vi "ISEG_HVBoardGUI.getStatus.vi"(2 "Numeric":dbl) -> (16 "s? t:f":T1 items=["ERROR"=-1, "OK"=0, "NOT_OK"=1])   [LabVIEW 2014, in "ISEG_HVBoardGUI.lvlib"]
uses:
  ISEG_HVBoardGUI.lvlib
  CSCore/CSApplicationBaseClasses/DeviceBase/DeviceBase.deviceState.ctl
  CSCore/CSApplicationBaseClasses/DeviceBase/DeviceBase.lvlib
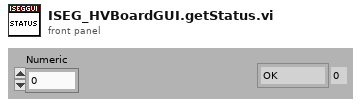
[diagram p1: front panel]
types:
  T1 = typedef "DeviceBase.lvlib/DeviceBase.deviceState.ctl" = i16
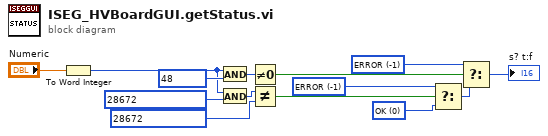
[diagram p0: block diagram]
diagram:
  w2 = T1 0 items=["ERROR"=-1, "OK"=0, "NOT_OK"=1] ("deviceState")
  w8 = T1 -1 items=["ERROR"=-1, "OK"=0, "NOT_OK"=1] ("deviceState")
  w3 = T1 -1 items=["ERROR"=-1, "OK"=0, "NOT_OK"=1] ("deviceState")
  n1 = To Word Integer(number="Numeric") -> (16bit integer=w4:i16)
  n2 = And(x=w4, y=i16 48) -> (x .and. y?=w13:i16)
  n3 = And(x=w4, y=i16 28672) -> (x .and. y?=w6:i16)
  n4 = Not Equal To 0?(x=w13) -> (x != 0?=w12:bool)
  n5 = Not Equal?(x=w6, y=i16 28672) -> (x != y?=w9:bool)
  n6 = Select(t=w8, s=w9, f=w2) -> (s? t:f=w7:T1)
  n7 = Select(t=w3, s=w12, f=w7) -> (s? t:f=→"s? t:f":T1)
